vi "FGV SPAN Verriegelung.vi"(2 "Processing Cluster":T6, 4 "Lin Param Elements Array":refnum<vi>[](array[refnum]), 5 "active SPAN Index":i32, 6 "aktion":T7, 7 "Component Cluster":T4={"Component"={"Component Name"="", "Component"=0, "Component Unit"=""}, "Daten aufzeichnen Offset Cluster"={"Autorange Offsets"="", "Autorange Spanfactors"="", "Polynome"={"Polynome[0]"=0.0, "Polynome[1]"=0.0, "Polynome[2]"=0.0, "Polynome[3]"=0.0, "Polynome[4]"=0.0}}, "Lin Offset Cluster"={"Autorange Offsets"="", "Autorange Spanfactors"="", "Polynome"={"Polynome[0]"=0.0, "Polynome[1]"=0.0, "Polynome[2]"=0.0, "Polynome[3]"=0.0, "Polynome[4]"=0.0}, "Polynom-Ordnung"=enum."autom."}, "EPA Optionsfeld"=enum."Rohwert"}, 8 "error in (no error)":errorcluster caption="Fehler (Eingang, kein Fehler)", 9 "Components Array":refnum<vi>[](array[refnum]), 10 "Buttons Array":refnum<vi>[](array[refnum]), 11 "Set Component Cluster":T5) -> (0 "error out":errorcluster caption="Fehler (Ausgang)", 1 "Flags Cluster":T1, 3 "locked":bool)   [LabVIEW 2020, in "Linearisierung v2.lvlib" / "SpanEinstellungen.lvlib"]
uses:
  SpanEinstellungen.lvlib
  Aktion FGV SPAN Verriegelung.ctl
  Auswahl Polynom Ordnung.ctl
  EPA Optionsfeld.ctl
  Linearisierung v2.lvlib
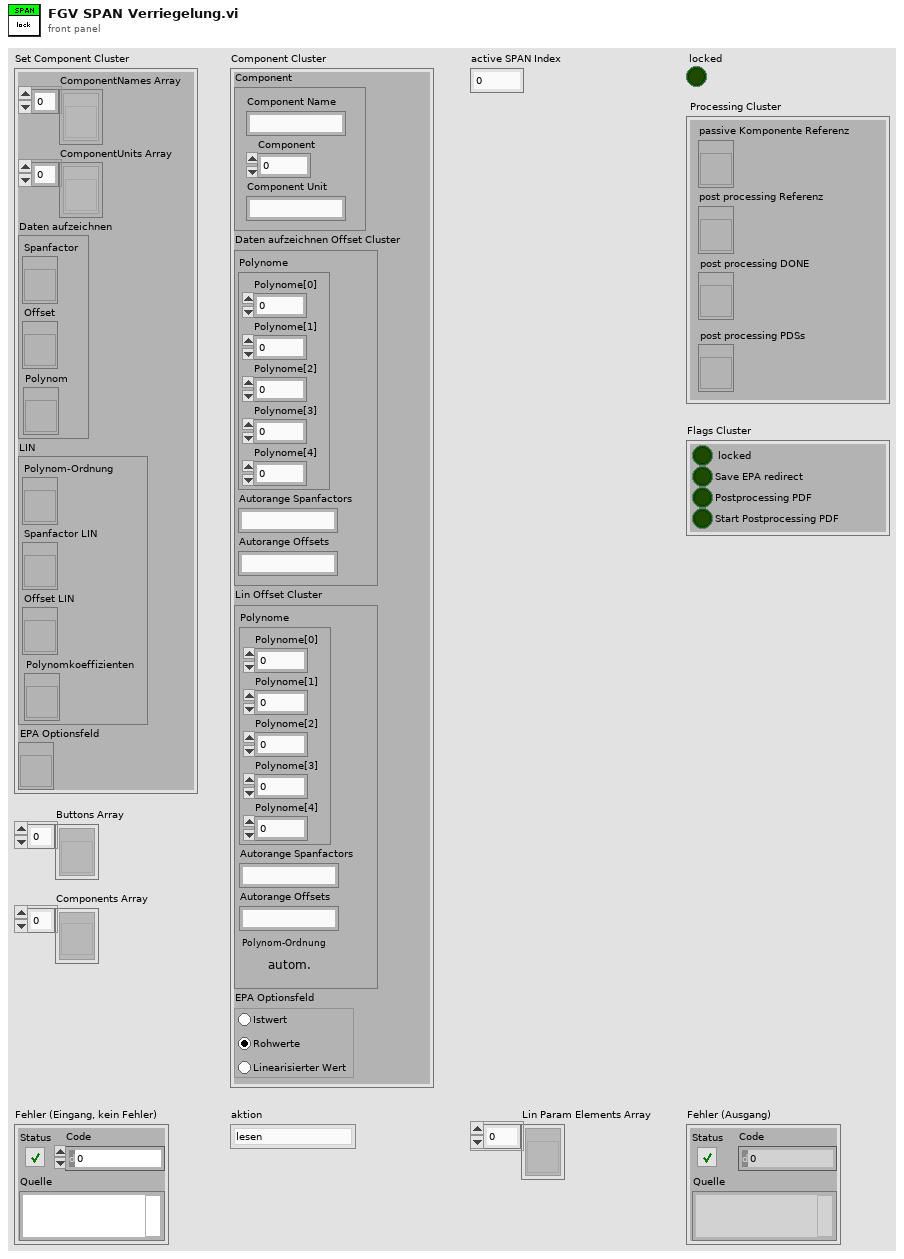
[diagram p1: front panel]
types:
  T1 = cluster{"locked":bool, "Save EPA redirect":bool, "Postprocessing PDF":bool, "Start Postprocessing PDF":bool}
  T2 = typedef "Linearisierung v2.lvlib/Auswahl Polynom Ordnung.ctl" = enum16{"autom.", "raw", "actual", "1", "2", "3", "4"}
  T3 = typedef "Linearisierung v2.lvlib/EPA Optionsfeld.ctl" = enum32{"Istwert", "Rohwert", "Linearisierter Wert"}
  T4 = cluster{"Component":cluster{"Component Name":string, "Component":u8, "Component Unit":string}, "Daten aufzeichnen Offset Cluster":cluster{"Autorange Offsets":string, "Autorange Spanfactors":string, "Polynome":cluster{"Polynome[0]":dbl, "Polynome[1]":dbl, "Polynome[2]":dbl, "Polynome[3]":dbl, "Polynome[4]":dbl}}, "Lin Offset Cluster":cluster{"Autorange Offsets":string, "Autorange Spanfactors":string, "Polynome":cluster{"Polynome[0]":dbl, "Polynome[1]":dbl, "Polynome[2]":dbl, "Polynome[3]":dbl, "Polynome[4]":dbl}, "Polynom-Ordnung":T2}, "EPA Optionsfeld":T3}
  T5 = cluster{"ComponentNames Array":refnum<vi>[], "ComponentUnits Array":refnum<vi>[], "Daten aufzeichnen":cluster{"Spanfactor":refnum<vi>, "Offset":refnum<vi>, "Polynom":refnum<vi>}, "LIN":cluster{"Polynom-Ordnung":refnum<vi>, "Spanfactor LIN":refnum<vi>, "Offset LIN":refnum<vi>, "Polynomkoeffizienten":refnum<vi>}, "EPA Optionsfeld":refnum<vi>}
  T6 = cluster{"passive Komponente Referenz":refnum<vi>, "post processing Referenz":refnum<vi>, "post processing DONE":refnum<vi>, "post processing PDSs":refnum<vi>}
  T7 = typedef "Linearisierung v2.lvlib/SpanEinstellungen.lvlib/Aktion FGV SPAN Verriegelung.ctl" = enum16{"lesen", "setrefs", "setcomp", "lock", "unlock", "Set Save EPA redirect", "Reset Save EPA redirect", "Set Postprocessing PDF", "Reset Postprocessing PDF", "Set Start Postprocessing PDF", "Reset Start Postprocessing PDF"}
  T8 = enum8{"Enabled", "Disabled", "Disabled and Grayed Out"}
  T9 = cluster{"Component Name":string, "Component":u8, "Component Unit":string}
  T10 = cluster{"Autorange Offsets":string, "Autorange Spanfactors":string, "Polynome":cluster{"Polynome[0]":dbl, "Polynome[1]":dbl, "Polynome[2]":dbl, "Polynome[3]":dbl, "Polynome[4]":dbl}}
  T11 = cluster{"Autorange Offsets":string, "Autorange Spanfactors":string, "Polynome":cluster{"Polynome[0]":dbl, "Polynome[1]":dbl, "Polynome[2]":dbl, "Polynome[3]":dbl, "Polynome[4]":dbl}, "Polynom-Ordnung":T2}
  T12 = cluster{"Spanfactor":refnum<vi>, "Offset":refnum<vi>, "Polynom":refnum<vi>}
  T13 = cluster{"Polynom-Ordnung":refnum<vi>, "Spanfactor LIN":refnum<vi>, "Offset LIN":refnum<vi>, "Polynomkoeffizienten":refnum<vi>}
  T14 = cluster{"locked":bool, "Save EPA redirect":bool, "Postprocessing PDF":bool, bool}
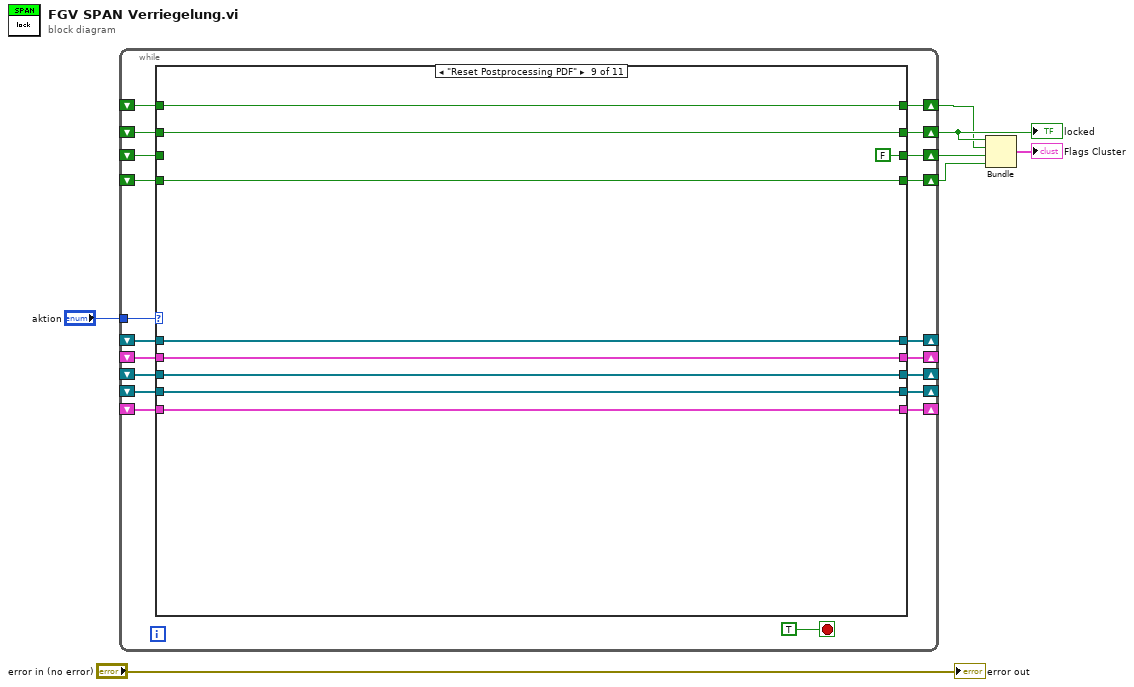
[diagram p0: block diagram]
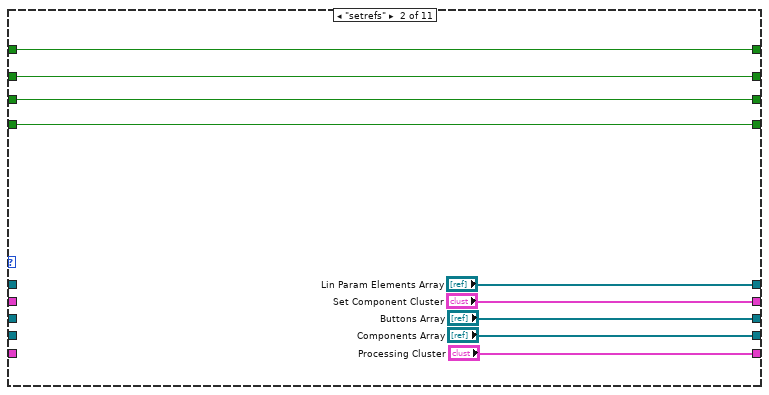
[diagram p3: hidden frame]
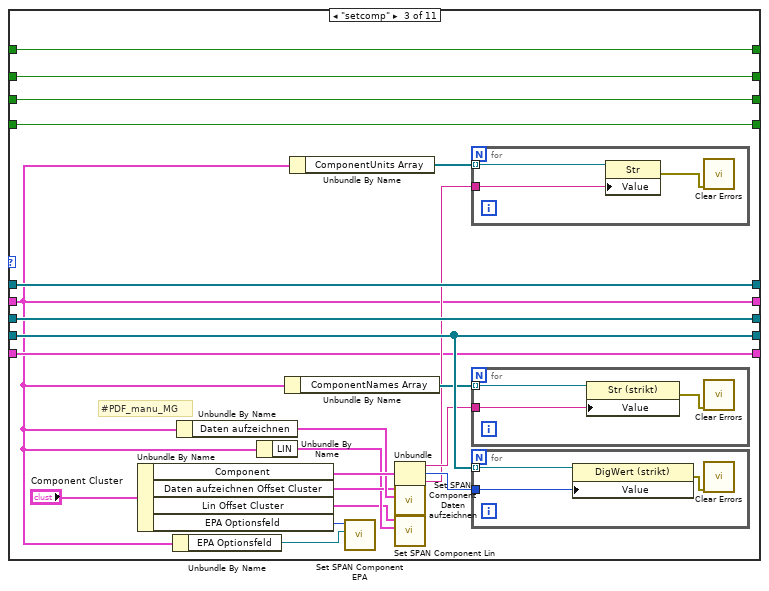
[diagram p4: hidden frame]
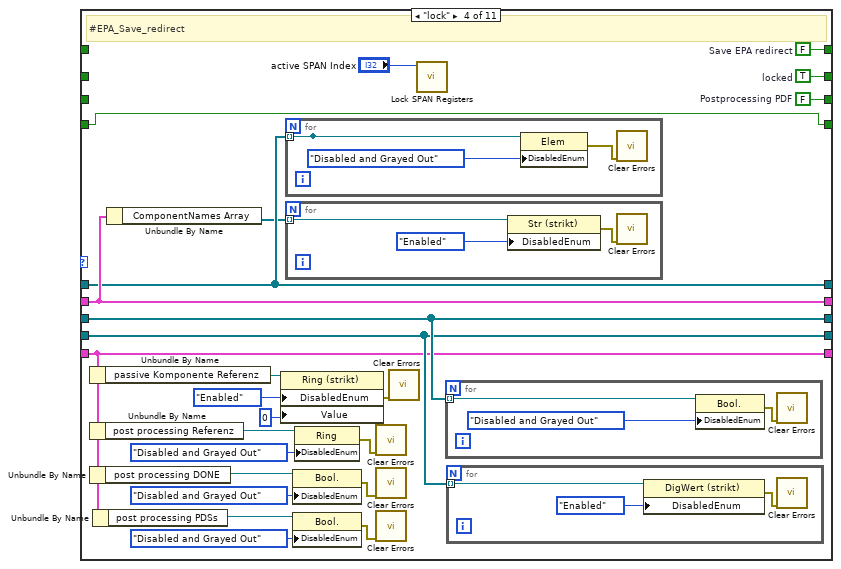
[diagram p5: hidden frame]
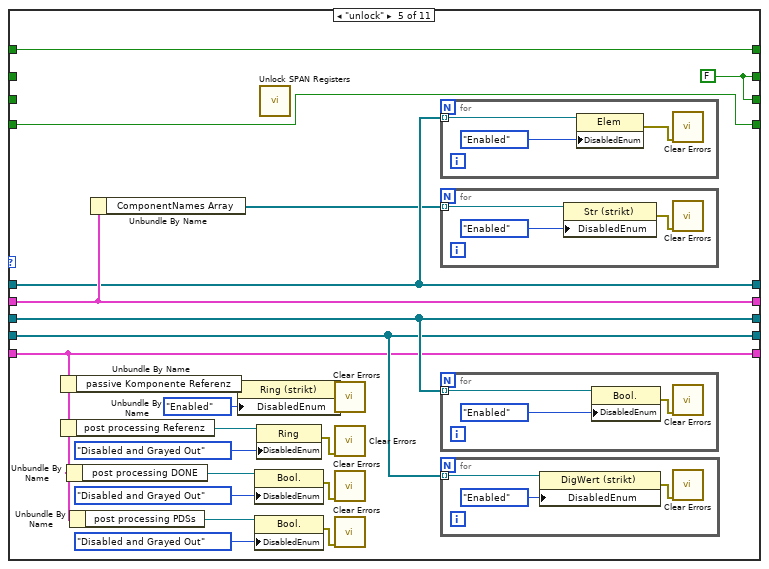
[diagram p6: hidden frame]
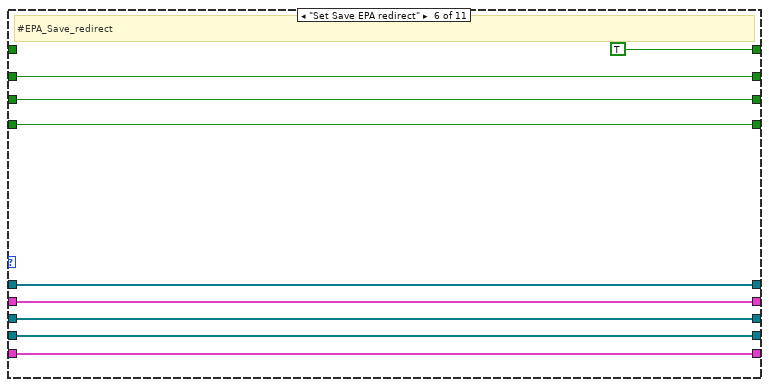
[diagram p7: hidden frame]
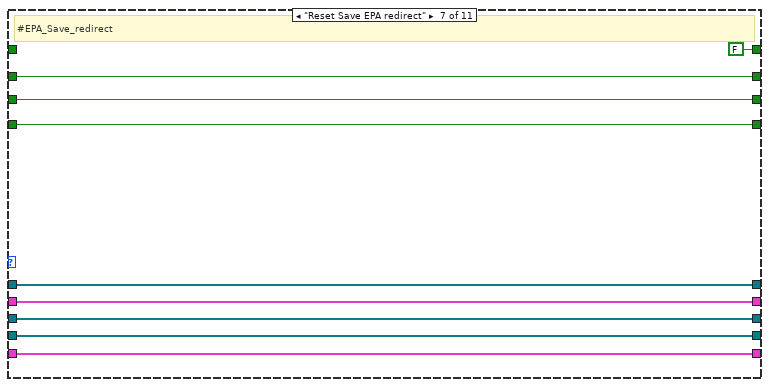
[diagram p8: hidden frame]
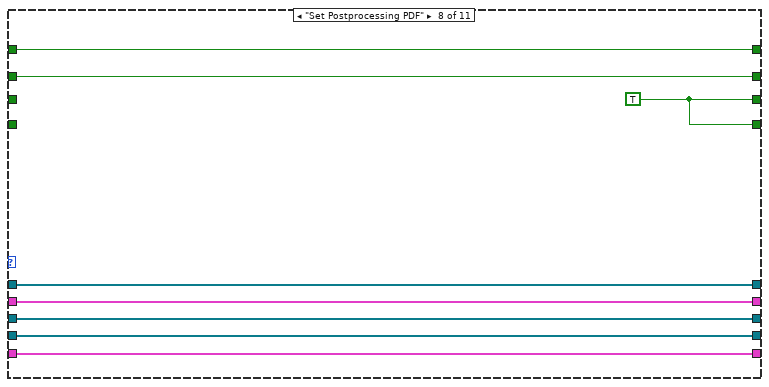
[diagram p9: hidden frame]
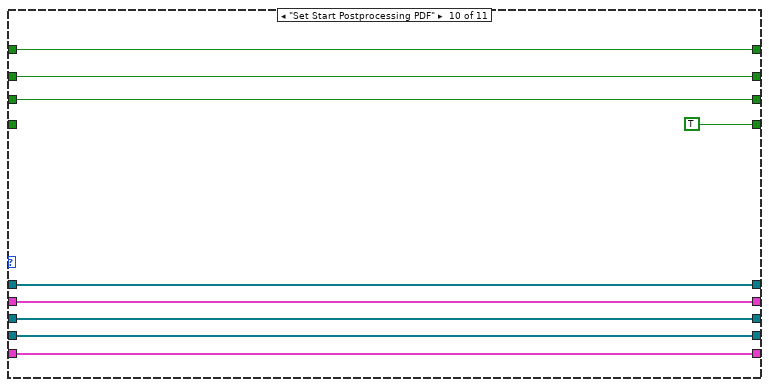
[diagram p10: hidden frame]
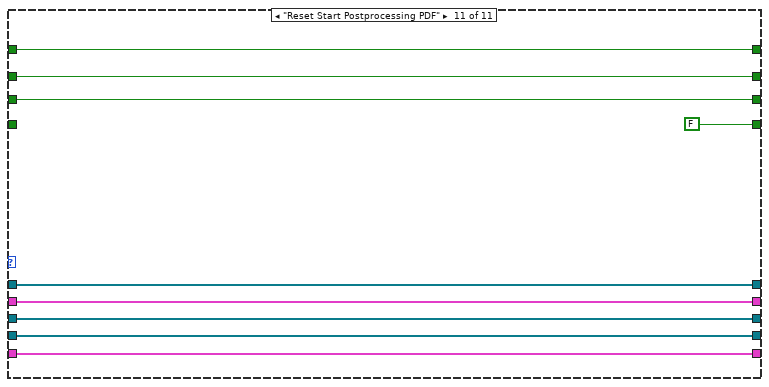
[diagram p11: hidden frame]
diagram:
  n1 = while {
    tunnel: "aktion" -> [w26]
    shift-right: [w25] -> _
    shift-left: _ -> [w22]
    shift-right: [w24] -> _
    shift-left: _ -> [w21]
    shift-right: [w23] -> _
    shift-left: _ -> [w20]
    shift-right: [w19] -> _
    shift-left: _ -> [w18]
    shift-right: [w17] -> w5
    shift-left: _ -> [w16]
    shift-right: [w15] -> _
    shift-left: _ -> [w14]
    shift-right: [w13] -> w4
    shift-left: _ -> [w12]
    shift-right: [w11] -> w3
    shift-left: _ -> [w10]
    shift-right: [w9] -> w1
    shift-left: _ -> [w8]
    stop <- TRUE stop-if-true
    n2 = case shown="\"Reset Postprocessing PDF\"" w26 {
      tunnel: [w36 "Set Component Cluster" w50 w97 w131 w154 w163 w171 w180 w189 w198] -> w25
      tunnel: [w35 "Buttons Array" w67 w100 w133 w153 w162 w170 w179 w188 w197] -> w24
      tunnel: [w34 "Components Array" w66 w99 w132 w152 w161 w169 w178 w187 w196] -> w23
      tunnel: w22 -> [w36 _ w50 w97 w131 w154 w163 w171 w180 w189 w198]
      tunnel: w21 -> [w35 _ w67 w100 w133 w153 w162 w170 w179 w188 w197]
      tunnel: w20 -> [w34 _ w66 w99 w132 w152 w161 w169 w178 w187 w196]
      tunnel: [w33 "Lin Param Elements Array" w63 w96 w130 w151 w160 w168 w177 w186 w195] -> w19
      tunnel: w18 -> [w33 _ w63 w96 w130 w151 w160 w168 w177 w186 w195]
      tunnel: [w32 w42 w62 w95 w114 w150 w159 w167 w176 w185 w194] -> w17
      tunnel: w16 -> [w32 w42 w62 _ _ w150 w159 w167 w176 w185 w194]
      tunnel: [w31 "Processing Cluster" w58 w79 w115 w149 w158 w166 w175 w184 w193] -> w15
      tunnel: w14 -> [w31 _ w58 w79 w115 w149 w158 w166 w175 w184 w193]
      tunnel: [w30 w39 w48 w83 w119 TRUE FALSE w165 w174 w183 w192] -> w13
      tunnel: w12 -> [w30 w39 w48 _ w119 _ _ w165 w174 w183 w192]
      tunnel: [w29 w38 w47 w78 w114 w147 w156 w164 FALSE w182 w191] -> w11
      tunnel: w10 -> [w29 w38 w47 _ _ w147 w156 _ _ w182 w191]
      tunnel: [w28 w37 w46 w77 w113 w146 w155 w164 w172 TRUE FALSE] -> w9
      tunnel: w8 -> [w28 w37 w46 w77 w113 w146 w155 _ w172 _ _]
      frame "lesen", Default {
      }
      frame "setrefs" {
      }
      frame "setcomp" {
        # "#PDF_manu_MG"
        n3 = Unbundle By Name("Component Cluster") -> ("Component"=w56:T9, "Daten aufzeichnen Offset Cluster"=w53:T10, "Lin Offset Cluster"=w51:T11, "EPA Optionsfeld"=w55:T3)
        n4 = Unbundle By Name(w50) -> ("EPA Optionsfeld"=w49:refnum<vi>)
        n5 = Unbundle By Name(w50) -> ("Daten aufzeichnen"=w54:T12)
        n6 = Unbundle By Name(w50) -> ("LIN"=w52:T13)
        n7 = Unbundle By Name(w50) -> ("ComponentNames Array"=w61:refnum<vi>[])
        n8 = Unbundle By Name(w50) -> ("ComponentUnits Array"=w60:refnum<vi>[])
        n9 = call "Set SPAN Component EPA.vi"(10:"EPA Optionsfeld"=w49, 11:"EPA Optionsfeld"=w55) -> ()  [unwired: 10 in]
        n10 = Unbundle(w56) -> ("Component Name"=w65:string, "Component"=w64:u8, "Component Unit"=w59:string)
        n11 = call "Set SPAN Component Daten aufzeichnen.vi"("Daten aufzeichnen"=w54, "Daten aufzeichnen Offset Cluster"=w53) -> ()  [unwired: 10 in]
        n12 = call "Set SPAN Component Lin.vi"("LIN"=w52, "Lin Offset Cluster"=w51) -> ()  [unwired: 10 in]
        n13 = for {
          tunnel: w60 -> [w70] mode=indexing
          tunnel: w59 -> [w68]
          n14 = property class="Str"(reference=w70, "Value"=w68) -> (error out=w69:errorcluster)  [unwired: 1 in, 1 out]
          n15 = call <vilib>:"Clear Errors.vi"("error in (no error)"=w69) -> ()  [unwired: 5 in, 2 out]
        }
        n16 = for {
          tunnel: w61 -> [w76] mode=indexing
          tunnel: w65 -> [w74]
          n17 = property class="Str (strikt)"(reference=w76, "Value"=w74) -> (error out=w75:errorcluster)  [unwired: 1 in, 1 out]
          n18 = call <vilib>:"Clear Errors.vi"("error in (no error)"=w75) -> ()  [unwired: 5 in, 2 out]
        }
        n19 = for {
          tunnel: w66 -> [w73] mode=indexing
          tunnel: w64 -> [w71]
          n20 = property class="DigWert (strikt)"(reference=w73, "Value"=w71) -> (error out=w72:errorcluster)  [unwired: 1 in, 1 out]
          n21 = call <vilib>:"Clear Errors.vi"("error in (no error)"=w72) -> ()  [unwired: 5 in, 2 out]
        }
      }
      frame "lock" {
        w78 = FALSE  # Postprocessing PDF
        w83 = FALSE  # Save EPA redirect
        w95 = TRUE  # locked
        # "#EPA_Save_redirect"
        n22 = Unbundle By Name(w79) -> ("passive Komponente Referenz"=w91:refnum<vi>)
        n23 = Unbundle By Name(w79) -> ("post processing Referenz"=w88:refnum<vi>)
        n24 = Unbundle By Name(w79) -> ("post processing DONE"=w87:refnum<vi>)
        n25 = Unbundle By Name(w79) -> ("post processing PDSs"=w80:refnum<vi>)
        n26 = Unbundle By Name(w97) -> ("ComponentNames Array"=w94:refnum<vi>[])
        n27 = property class="Ring (strikt)"(reference=w91, "DisabledEnum"=T8."Enabled" ("Deaktiviert"), "Value"=u16 0 ("Wert")) -> (error out=w92:errorcluster)  [unwired: 1 in, 1 out]
        n28 = for {
          tunnel: [w101] -> _ mode=indexing
          tunnel: w96 -> [w101] mode=indexing
          n29 = property class="Elem"(reference=w101, "DisabledEnum"=T8."Disabled and Grayed Out" ("Deaktiviert")) -> (error out=w102:errorcluster)  [unwired: 1 in, 1 out]
          n30 = call <vilib>:"Clear Errors.vi"("error in (no error)"=w102) -> ()  [unwired: 5 in, 2 out]
        }
        n31 = for {
          tunnel: w94 -> [w106] mode=indexing
          n32 = property class="Str (strikt)"(reference=w106, "DisabledEnum"=T8."Enabled" ("Deaktiviert")) -> (error out=w104:errorcluster)  [unwired: 1 in, 1 out]
          n33 = call <vilib>:"Clear Errors.vi"("error in (no error)"=w104) -> ()  [unwired: 5 in, 2 out]
        }
        n34 = property class="Bool."(reference=w87, "DisabledEnum"=T8."Disabled and Grayed Out" ("Deaktiviert")) -> (error out=w86:errorcluster)  [unwired: 1 in, 1 out]
        n35 = property class="Bool."(reference=w80, "DisabledEnum"=T8."Disabled and Grayed Out" ("Deaktiviert")) -> (error out=w81:errorcluster)  [unwired: 1 in, 1 out]
        n36 = property class="Ring"(reference=w88, "DisabledEnum"=T8."Disabled and Grayed Out" ("Deaktiviert")) -> (error out=w90:errorcluster)  [unwired: 1 in, 1 out]
        n37 = call <vilib>:"Clear Errors.vi"("error in (no error)"=w90) -> ()  [unwired: 5 in, 2 out]
        n38 = call <vilib>:"Clear Errors.vi"("error in (no error)"=w86) -> ()  [unwired: 5 in, 2 out]
        n39 = call <vilib>:"Clear Errors.vi"("error in (no error)"=w81) -> ()  [unwired: 5 in, 2 out]
        n40 = call <vilib>:"Clear Errors.vi"("error in (no error)"=w92) -> ()  [unwired: 5 in, 2 out]
        n41 = call "Lock SPAN Registers.vi"("active SPAN Index"="active SPAN Index") -> ()  [unwired: 10 in, 1 out]
        n42 = for {
          tunnel: w100 -> [w112] mode=indexing
          n43 = property class="Bool."(reference=w112, "DisabledEnum"=T8."Disabled and Grayed Out" ("Deaktiviert")) -> (error out=w110:errorcluster)  [unwired: 1 in, 1 out]
          n44 = call <vilib>:"Clear Errors.vi"("error in (no error)"=w110) -> ()  [unwired: 5 in, 2 out]
        }
        n45 = for {
          tunnel: w99 -> [w109] mode=indexing
          n46 = property class="DigWert (strikt)"(reference=w109, "DisabledEnum"=T8."Enabled" ("Deaktiviert")) -> (error out=w107:errorcluster)  [unwired: 1 in, 1 out]
          n47 = call <vilib>:"Clear Errors.vi"("error in (no error)"=w107) -> ()  [unwired: 5 in, 2 out]
        }
      }
      frame "unlock" {
        w114 = FALSE
        n48 = Unbundle By Name(w115) -> ("passive Komponente Referenz"=w126:refnum<vi>)
        n49 = Unbundle By Name(w115) -> ("post processing Referenz"=w125:refnum<vi>)
        n50 = Unbundle By Name(w115) -> ("post processing DONE"=w120:refnum<vi>)
        n51 = Unbundle By Name(w115) -> ("post processing PDSs"=w118:refnum<vi>)
        n52 = Unbundle By Name(w131) -> ("ComponentNames Array"=w129:refnum<vi>[])
        n53 = property class="Ring (strikt)"(reference=w126, "DisabledEnum"=T8."Enabled" ("Deaktiviert")) -> (error out=w127:errorcluster)  [unwired: 1 in, 1 out]
        n54 = property class="Bool."(reference=w120, "DisabledEnum"=T8."Disabled and Grayed Out" ("Deaktiviert")) -> (error out=w121:errorcluster)  [unwired: 1 in, 1 out]
        n55 = property class="Bool."(reference=w118, "DisabledEnum"=T8."Disabled and Grayed Out" ("Deaktiviert")) -> (error out=w117:errorcluster)  [unwired: 1 in, 1 out]
        n56 = property class="Ring"(reference=w125, "DisabledEnum"=T8."Disabled and Grayed Out" ("Deaktiviert")) -> (error out=w124:errorcluster)  [unwired: 1 in, 1 out]
        n57 = call "Unlock SPAN Registers.vi"() -> ()  [unwired: 11 in, 1 out]
        n58 = call <vilib>:"Clear Errors.vi"("error in (no error)"=w127) -> ()  [unwired: 5 in, 2 out]
        n59 = call <vilib>:"Clear Errors.vi"("error in (no error)"=w124) -> ()  [unwired: 5 in, 2 out]
        n60 = call <vilib>:"Clear Errors.vi"("error in (no error)"=w121) -> ()  [unwired: 5 in, 2 out]
        n61 = call <vilib>:"Clear Errors.vi"("error in (no error)"=w117) -> ()  [unwired: 5 in, 2 out]
        n62 = for {
          tunnel: w130 -> [w136] mode=indexing
          n63 = property class="Elem"(reference=w136, "DisabledEnum"=T8."Enabled" ("Deaktiviert")) -> (error out=w134:errorcluster)  [unwired: 1 in, 1 out]
          n64 = call <vilib>:"Clear Errors.vi"("error in (no error)"=w134) -> ()  [unwired: 5 in, 2 out]
        }
        n65 = for {
          tunnel: w129 -> [w139] mode=indexing
          n66 = property class="Str (strikt)"(reference=w139, "DisabledEnum"=T8."Enabled" ("Deaktiviert")) -> (error out=w137:errorcluster)  [unwired: 1 in, 1 out]
          n67 = call <vilib>:"Clear Errors.vi"("error in (no error)"=w137) -> ()  [unwired: 5 in, 2 out]
        }
        n68 = for {
          tunnel: w133 -> [w145] mode=indexing
          n69 = property class="Bool."(reference=w145, "DisabledEnum"=T8."Enabled" ("Deaktiviert")) -> (error out=w143:errorcluster)  [unwired: 1 in, 1 out]
          n70 = call <vilib>:"Clear Errors.vi"("error in (no error)"=w143) -> ()  [unwired: 5 in, 2 out]
        }
        n71 = for {
          tunnel: w132 -> [w142] mode=indexing
          n72 = property class="DigWert (strikt)"(reference=w142, "DisabledEnum"=T8."Enabled" ("Deaktiviert")) -> (error out=w140:errorcluster)  [unwired: 1 in, 1 out]
          n73 = call <vilib>:"Clear Errors.vi"("error in (no error)"=w140) -> ()  [unwired: 5 in, 2 out]
        }
      }
      frame "Set Save EPA redirect" {
        # "#EPA_Save_redirect"
      }
      frame "Reset Save EPA redirect" {
        # "#EPA_Save_redirect"
      }
      frame "Set Postprocessing PDF" {
        w164 = TRUE
      }
      frame "Reset Postprocessing PDF" {
      }
      frame "Set Start Postprocessing PDF" {
      }
      frame "Reset Start Postprocessing PDF" {
      }
    }
  }
  "locked" <- w5
  n74 = Bundle("locked"=w5, "Save EPA redirect"=w4, "Postprocessing PDF"=w3, w1) -> (→"Flags Cluster":T14)  [unwired: 1 in]
  "error out" <- "error in (no error)"
